vi "UMLEditor Main.vi"(1 "StartProject":string, 3 "StartTarget":string) -> ()   [LabVIEW 2012] (continued)
                        n1583 = call-dynamic "getBounds.vi"("reference"=w4053, "error in (no error)"=w4050) -> ("bounds"=w4048:T13, "error out"=w4051:errorcluster)  [unwired: 15 in, 1 out]
                        n1584 = Build Array(w4053) -> (w4047:refnum<class "AbstractNode.lvclass">[])
                        n1585 = Bundle By Name(cluster=w4055, "selcted"=UMLEditor_tooltype."Node", "SelectedNodes"=w4047, "dragStartBounds"=w4048, "dragStartPoint"=w4052, "lastMousePoint"=w4052, "newSelected"=TRUE, "toolType"=UMLEditor_tooltype."None", "tool"=UMLEditor_toolsType."CD_Select") -> (w4054:T7)
                        n1586 = call <resource>:"UMLEditor UpdatesToolbuttons.vi"() -> ()  [unwired: 6 in, 14 out]
                      }
                    }
                  }
                  frame True {
                    # "Added"
                    n1587 = case shown="\"AddNodeFromProjectTree+SyncAll\"" w4059 {
                      tunnel: [UMLEditor_statesType."Repaint" ("state") UMLEditor_statesType."SyncAll" ("state")] -> w4066
                      frame "AddNodeFromProjectTree", Default {
                      }
                      frame "AddNodeFromProjectTree+SyncAll" {
                      }
                    }
                    n1588 = To More Specific Class(target class=refnum<class "ClassNode.lvclass"> refnum ("reference"), reference=w4057) -> (specific class reference=w4056:refnum<class "ClassNode.lvclass">)  [unwired: 1 in, 1 out]
                    n1589 = call-dynamic "ExternalSetParam.vi"("reference"=w4056, "setParameter"=ExternalSetTypes."Name", "string"=w4067, "error in (no error)"=w4069) -> ("reference out"=w4063:refnum<class "ClassNode.lvclass">, "error out"=w4065:errorcluster)  [unwired: 14 in]
                    n1590 = call-dynamic "ExternalSetParam.vi"("reference"=w4063, "setParameter"=ExternalSetTypes."ClassPath", "error in (no error)"=w4065, "ClassPath"=w4060) -> ("reference out"=w4062:refnum<class "ClassNode.lvclass">, "error out"=w4064:errorcluster)  [unwired: 14 in]
                    n1591 = call-dynamic "getBounds.vi"("reference"=w4062, "error in (no error)"=w4064) -> ("reference out"=w4079:refnum<class "ClassNode.lvclass">, "bounds"=w4080:T13, "error out"=w4076:errorcluster)  [unwired: 15 in]
                    n1592 = Build Array(w4079) -> (w4071:refnum<class "ClassNode.lvclass">[])
                    n1593 = Bundle By Name(cluster=w4074, "selcted"=UMLEditor_tooltype."Node", "SelectedNodes"=w4071, "dragStartBounds"=w4080, "dragStartPoint"=w4070, "lastMousePoint"=w4070) -> (w4073:T7)
                    n1594 = call <resource>:"UMLEditor setDiagramInfo.vi"("error in (no error)"=w4076, "localVariablesIn"=w4073, "action"=enum16{"Name/Dir", "Unsaved", "Saved"}."Unsaved") -> ("localVariablesOut"=w4072:T7, "error out"=w4075:errorcluster)  [unwired: 2 in, 13 out]
                  }
                }
              }
            }
            n1595 = for {
              tunnel: w3971 -> [_]
              tunnel: w3946 -> [w4095] mode=indexing
              tunnel: [w4094] -> _
              n1596 = Close Reference(reference=w4095) -> (error out=w4094:errorcluster)  [unwired: 1 in]
            }
          }
          frame True {
            n1597 = call <resource>:"GDSError_ClearError.vi"("code"=1055, "error in (no error)"=w4098) -> ("error out"=w4097:errorcluster)  [unwired: 3 in, 14 out]
          }
        }
      }
      frame "AnalyseViInStateDiagram" {
        n1598 = Unbundle By Name(w4105) -> ("diagrams"=w4127:T39)
        n1599 = Unbundle By Name(w4105) -> ("menu"=w4120:refnum<k9>, "Action"=w4104:string)
        n1600 = property on="toolTab" class="TabCtl (strict)"("Disabled"=u8 0) -> ()  [unwired: 2 in, 2 out]
        n1601 = local write "Diagram"(0) -> ()
        n1602 = call <resource>:"UMLEditor UpdatesToolbuttons.vi"() -> ()  [unwired: 6 in, 14 out]
        n1603 = for {
          tunnel: w4127 -> [w4190] mode=indexing
          tunnel: "Untitled %d" -> [w4188]
          tunnel: [w4187] -> w4125 mode=indexing
          n1604 = Unbundle By Name(w4190) -> ("name"=w4189:string)
          n1605 = Scan From String(format string=w4188, input string=w4189) -> (output 1=w4187:i32)  [unwired: 2 in, 4 out]
        }
        n1606 = String To Path(string=w4104) -> (path=w4103:path)
        n1607 = Bundle By Name(cluster=T32 {"VI-Path"=path "", "ShowOption"=enum."Show Relative Path"} ("StateDiagramData"), "VI-Path"=w4103) -> (w4110:T32)
        n1608 = Unbundle By Name(w4105) -> ("grid"=w4112:refnum<class "Grid.lvclass">, "graphics"=w4111:refnum<class "Graphics.lvclass">)
        n1609 = Array Max & Min(array=w4125) -> (max value=w4124:i32)  [unwired: 3 out]
        n1610 = call <resource>:"StateDiagramGraph_Create.vi"("StateDiagramData"=w4110, "error in (no error)"=w4109) -> ("reference out"=w4115:refnum<class "StateDiagramGraph.lvclass">, "error out"=w4114:errorcluster)  [unwired: 2 in, 14 out]
        n1611 = property on="Picture" class="Pict"() -> (error out=w4102:errorcluster, "Visible"=w4101:bool)  [unwired: 2 in, 1 out]
        n1612 = call-dynamic "HandleRightClickMenuOption.vi"("reference"=w4115, "MenuOption"="Create New Diagram", "graphics"=w4111, "grid"=w4112, "error in (no error)"=w4114) -> ("reference out"=w4108:refnum<class "StateDiagramGraph.lvclass">, "Cancel"=w4107:bool, "error out"=w4106:errorcluster)  [unwired: 12 in]
        n1613 = property on="Picture" class="Pict"(error in=w4102, "Visible"=TRUE) -> ()  [unwired: 1 in, 2 out]
        n1614 = case shown="False" w4107 {
          tunnel: w4124 -> [w4153 _]
          tunnel: w4120 -> [w4135 _]
          tunnel: [w4134 w4184] -> w4119
          tunnel: [w4133 w4183] -> w4118
          tunnel: w4105 -> [w4132 w4183]
          tunnel: [UMLEditor_statesType."Repaint" ("state") UMLEditor_statesType."Idle" ("state")] -> w4117
          tunnel: w4108 -> [w4129 w4185]
          tunnel: w4106 -> [w4128 w4186]
          tunnel: w4101 -> [_ w4181]
          frame False {
            w4144 = diagramType."State" ("diagramType")
            n1615 = Increment(x=w4153) -> (x+1=w4151:i32)
            n1616 = local read "Help"() -> (w4145:bool)
            n1617 = Format Into String(format string="Untitled %d", w4151) -> (resulting string=w4147:string)  [unwired: 2 in, 1 out]
            n1618 = property on="Diagram" class="Ring (strict)"("Tip Strip"=w4147) -> ()  [unwired: 2 in, 2 out]
            n1619 = case shown="True" w4145 {
              tunnel: w4144 -> [_ w4157]
              frame False {
              }
              frame True {
                n1620 = case shown="\"State\"" w4157 {
                  tunnel: [ContextHelp_HelpTexts."ClassDiagram_Help" ("HelpText") ContextHelp_HelpTexts."UseCaseDiagram_Help" ("HelpText") ContextHelp_HelpTexts."SequenceDiagram_Help" ("HelpText") ContextHelp_HelpTexts."StateDiagram_Help" ("HelpText")] -> w4155
                  frame "Class", Default {
                  }
                  frame "UseCase" {
                  }
                  frame "Sequency" {
                  }
                  frame "State" {
                  }
                }
                n1621 = call <resource>:"ContextHelp_HelpTexts.vi"("HelpText (enum or string)"=w4155) -> ("HelpOut"=w4156:T57)  [unwired: 18 out]
                n1622 = call <resource>:"ContextHelp_SendMessageToPopUp.vi"("PopUpMessage"=w4156) -> ()  [unwired: 2 in, 17 out]
              }
            }
            n1623 = call <resource>:"UndoEngine.vi"("reference"=w4129, "Action"=enum16{"TakeSnapshot", "Undo", "Redo"}."TakeSnapshot", "Reset"=TRUE, "error in (no error)"=w4128, "menu"=w4135) -> ("error out"=w4130:errorcluster)  [unwired: 3 in, 11 out]
            n1624 = call <resource>:"UMLEditor addDiagram.vi"("graph"=w4129, "diagramType"=w4144, "name"=w4147, "saveDir"=path "", "unsaved(False)"=FALSE, "error in (no error)"=w4130, "localVariablesIn"=w4132) -> ("localVariablesOut"=w4148:T7, "error out"=w4149:errorcluster)  [unwired: 11 out]
            n1625 = case shown="\"Class\", Default" w4144 {
              tunnel: w4148 -> [w4163 w4167 w4171 w4176 w4180]
              tunnel: [w4162 w4166 w4170 w4175 w4179] -> w4142
              frame "None" {
                n1626 = Bundle By Name(cluster=w4163, "tool"=UMLEditor_toolsType."CD_Select") -> (w4162:T7)
              }
              frame "Sequency" {
                n1627 = property on="toolTab" class="TabCtl (strict)"("Value"=enum32{"Class", "Sequence", "UseCase"}."Sequence" ("toolTab")) -> ()  [unwired: 2 in, 2 out]
                n1628 = Bundle By Name(cluster=w4167, "tool"=UMLEditor_toolsType."SQD_Select") -> (w4166:T7)
              }
              frame "UseCase" {
                n1629 = property on="toolTab" class="TabCtl (strict)"("Value"=enum32{"Class", "Sequence", "UseCase"}."UseCase" ("toolTab")) -> ()  [unwired: 2 in, 2 out]
                n1630 = Bundle By Name(cluster=w4171, "tool"=UMLEditor_toolsType."UD_Select") -> (w4170:T7)
              }
              frame "State" {
                n1631 = property on="toolTab" class="TabCtl (strict)"("Value"=enum32{"Class", "Sequence", "UseCase", "State"}."State" ("toolTab")) -> ()  [unwired: 2 in, 2 out]
                n1632 = Bundle By Name(cluster=w4176, "tool"=UMLEditor_toolsType."STD_Select") -> (w4175:T7)
              }
              frame "Class", Default {
                n1633 = Bundle By Name(cluster=w4180, "tool"=UMLEditor_toolsType."CD_Select") -> (w4179:T7)
                n1634 = property on="toolTab" class="TabCtl (strict)"("Value"=enum32{"Class", "Sequence", "UseCase"}."Class" ("toolTab")) -> ()  [unwired: 2 in, 2 out]
              }
            }
            n1635 = Unbundle By Name(w4132) -> ("menu"=w4143:refnum<k9>)
            n1636 = Bundle By Name(cluster=w4142, "selectedEdge"=refnum<class "AbstractEdge.lvclass"> refnum, "SelectedNodes"=refnum<class "AbstractNode.lvclass">[] [], "selcted"=UMLEditor_tooltype."None", "toolType"=UMLEditor_tooltype."None") -> (w4133:T7)
            n1637 = call <resource>:"UMLEditor menuUpdates.vi"("menu"=w4143, "menuAction"=UMLEditor_MenuActionType."EnableSave", "error in (no error)"=w4149) -> ("error out"=w4134:errorcluster)  [unwired: 3 in, 13 out]
          }
          frame True {
            n1638 = property on="Picture" class="Pict"("Visible"=w4181) -> ()  [unwired: 2 in, 2 out]
            n1639 = call-dynamic "Destroy.vi"("reference"=w4185, "error in (no error)"=w4186) -> ("error out"=w4184:errorcluster)  [unwired: 16 in, 1 out]
          }
        }
      }
      frame "Copy", "CopyPaste" {
        n1640 = Unbundle By Name(w4192) -> ("SelectedNodes"=w4193:refnum<class "AbstractNode.lvclass">[], "menu"=w4196:refnum<k9>)
        n1641 = Array Size(array=w4193) -> (size(s)=w4197:i32)
        n1642 = case shown="1.." w4197 {
          tunnel: w4196 -> [_ w4213]
          tunnel: w4195 -> [w4201 w4205]
          tunnel: [w4201 w4206] -> w4194
          tunnel: w4193 -> [_ w4207]
          tunnel: w4192 -> [_ w4202]
          frame 0, Default {
          }
          frame 1.. {
            n1643 = call <resource>:"UMLEditor getDiagramInfo.vi"("localVariables"=w4202, "error in (no error)"=w4205) -> ("graph"=w4203:refnum<class "Graph.lvclass">, "error out"=w4204:errorcluster)  [unwired: 16 out]
            n1644 = call <resource>:"UMLEditor menuUpdates.vi"("menu"=w4213, "menuAction"=UMLEditor_MenuActionType."EnablePaste", "error in (no error)"=w4204) -> ("error out"=w4211:errorcluster)  [unwired: 3 in, 13 out]
            n1645 = call <resource>:"UMLEditor ClipBoard.vi"("menuAction"=UMLEditor_ClipBoardActionType."EmptyClipBoard", "error in (no error)"=w4211) -> ("error out"=w4209:errorcluster)  [unwired: 4 in, 13 out]
            n1646 = call <resource>:"UMLEditor ClipBoard.vi"("menuAction"=UMLEditor_ClipBoardActionType."InsertToClipBoard", "SelectedNodes"=w4207, "Graph"=w4203, "error in (no error)"=w4209) -> ("error out"=w4206:errorcluster)  [unwired: 2 in, 13 out]
          }
        }
        n1647 = case shown="\"CopyPaste\"" w4191 {
          tunnel: [UMLEditor_statesType."Paste" ("state") UMLEditor_statesType."Idle" ("state")] -> w4198
          frame "CopyPaste" {
          }
          frame Default {
          }
        }
      }
      frame "Paste" {
        n1648 = Unbundle By Name(w4215) -> ("graphics"=w4220:refnum<class "Graphics.lvclass">, "offset"=w4222:T12, "zoom"=w4221:dbl)
        n1649 = call <resource>:"UMLEditor getDiagramInfo.vi"("localVariables"=w4215, "error in (no error)"=w4219) -> ("graph"=w4216:refnum<class "Graph.lvclass">, "diagramType"=w4217:T11, "error out"=w4218:errorcluster)  [unwired: 15 out]
        n1650 = case shown="Default" w4217 {
          tunnel: [w4226 w4248] -> w4223
          tunnel: w4222 -> [_ w4245]
          tunnel: w4221 -> [_ w4244]
          tunnel: w4220 -> [_ w4243]
          tunnel: w4218 -> [w4226 w4235]
          tunnel: w4216 -> [_ w4234]
          tunnel: w4215 -> [w4225 w4233]
          tunnel: [w4225 w4232] -> w4214
          frame "None" {
          }
          frame Default {
            w4242 = cluster{dbl, dbl} {0.0, 0.0} ("lower limit")
            n1651 = property on="Picture" class="Pict"() -> ("Mouse"=w4237:T42)  [unwired: 2 in, 2 out]
            n1652 = Unbundle By Name(w4237) -> ("Mouse Position"=w4247:cluster{"X":i32, "Y":i32})
            n1653 = Add(x=w4247, y=w4245) -> (x+y=w4246:T12)
            n1654 = Divide(x=w4246, y=w4244) -> (x/y=w4228:T12)
            n1655 = call <resource>:"getScreenBounds.vi"("reference"=w4243, "error in (no error)"=w4235) -> ("bounds"=w4241:T13, "error out"=w4236:errorcluster)  [unwired: 16 out]
            n1656 = Unbundle By Name(w4241) -> ("width"=w4240:dbl, "height"=w4239:dbl)
            n1657 = Bundle(cluster=w4242, w4240, w4239) -> ()  [unwired: 1 out]
            n1658 = In Range and Coerce(upper limit=w4228, x=w4228, lower limit=w4242) -> (coerced(x)=w4238:T12)  [unwired: 1 out]
            n1659 = call <resource>:"UMLEditor ClipBoard.vi"("menuAction"=UMLEditor_ClipBoardActionType."PasteContentAtPos", "Pos"=w4238, "Graph"=w4234, "error in (no error)"=w4236, "LimitPasteToAllowedLocations(True)"=FALSE) -> ("PastedNodes"=w4231:refnum<class "AbstractNode.lvclass">[], "error out"=w4248:errorcluster)  [unwired: 2 in, 11 out]
            n1660 = Array Size(array=w4231) -> (size(s)=w4229:i32)
            n1661 = case shown="0" w4229 {
              tunnel: [UMLEditor_tooltype."Node" ("selcted") UMLEditor_tooltype."None" ("selcted")] -> w4230
              frame Default {
              }
              frame 0 {
              }
            }
            n1662 = Bundle By Name(cluster=w4233, "selcted"=w4230, "SelectedNodes"=w4231) -> (w4232:T7)
          }
        }
      }
      frame "Export" {
        w4253 = 0.0 ("y")
        w4252 = 5.0  # borderRoundPicture
        w4287 = 1.0 ("scaleX")
        n1663 = Unbundle By Name(w4260) -> ("graphics"=w4290:refnum<class "Graphics.lvclass">)
        n1664 = Unbundle By Name(w4260) -> ("exportype"=w4259:T14)
        n1665 = Unbundle By Name(w4260) -> ("grid"=w4282:refnum<class "Grid.lvclass">)
        n1666 = call-dynamic "clone.vi"("reference"=w4290, "error in (no error)"=w4289) -> ("clonedObjectRef"=w4288:refnum<class "Graphics.lvclass">, "error out"=w4286:errorcluster)  [unwired: 15 in, 1 out]
        n1667 = call <resource>:"scale.vi"("reference"=w4288, "scaleX"=w4287, "scaleY"=w4287, "error in (no error)"=w4286) -> ("reference out"=w4278:refnum<class "Graphics.lvclass">, "error out"=w4279:errorcluster)  [unwired: 14 out]
        n1668 = call <resource>:"resetPicture.vi"("reference"=w4278, "error in (no error)"=w4279) -> ("reference out"=w4277:refnum<class "Graphics.lvclass">, "error out"=w4276:errorcluster)  [unwired: 16 out]
        n1669 = call <resource>:"UMLEditor getDiagramInfo.vi"("localVariables"=w4260, "error in (no error)"=w4276) -> ("graph"=w4284:refnum<class "Graph.lvclass">, "name"=w4257:string, "saveDir"=w4258:path, "error out"=w4285:errorcluster)  [unwired: 14 out]
        n1670 = call-dynamic "getBounds.vi"("reference"=w4284, "graphics"=w4277, "error in (no error)"=w4285) -> ("reference out"=w4283:refnum<class "Graph.lvclass">, "bounds"=w4270:T13, "error out"=w4275:errorcluster)  [unwired: 14 in]
        n1671 = Unbundle By Name(w4270) -> ("width"=w4268:dbl, "height"=w4269:dbl)
        n1672 = Unbundle By Name(w4270) -> ("x"=w4274:dbl, "y"=w4271:dbl)
        n1673 = Subtract(x=w4274, y=w4253) -> (x-y=w4273:dbl)
        n1674 = Subtract(x=w4271, y=w4253) -> (x-y=w4272:dbl)
        n1675 = Add(x=w4268, y=w4269) -> (x+y=w4267:dbl)
        n1676 = Greater Than 0?(x=w4267) -> (x > 0?=w4266:bool)
        n1677 = call <resource>:"setOffset.vi"("reference"=w4277, "offsetX"=w4273, "offsetY"=w4272, "error in (no error)"=w4275) -> ("reference out"=w4265:refnum<class "Graphics.lvclass">, "error out"=w4254:errorcluster)  [unwired: 14 out]
        n1678 = Multiply(x=w4252, y=2.0) -> (x*y=w4261:dbl)
        n1679 = call-dynamic "draw.vi"("reference"=w4283, "graphics"=w4265, "grid"=w4282, "error in (no error)"=w4254, "SelectedNodes"=refnum<class "AbstractNode.lvclass">[] [], "HideOverLays(False)"=TRUE) -> ("NodesBounds"=w4281:T13, "error out"=w4263:errorcluster)  [unwired: 10 in, 2 out]
        n1680 = case shown="True" w4266 {
          tunnel: w4281 -> [_ _]
          tunnel: w4270 -> [_ w4314]
          tunnel: w4265 -> [_ w4315]
          tunnel: w4263 -> [w4292 w4300]
          tunnel: [w4292 w4300] -> w4264
          tunnel: w4261 -> [_ w4304]
          tunnel: w4259 -> [_ w4299]
          tunnel: w4259 -> [_ w4307]
          tunnel: w4258 -> [_ w4306]
          tunnel: w4257 -> [_ w4301]
          tunnel: w4252 -> [_ w4294]
          frame False {
          }
          frame True {
            n1681 = Match Pattern(string=w4301, regular expression="[.][~.]+$") -> (before substring=w4302:string)  [unwired: 4 out]
            n1682 = Unbundle By Name(w4314) -> ("x"=w4297:dbl, "y"=w4295:dbl, "width"=w4312:dbl, "height"=w4310:dbl)
            n1683 = case shown="\"None\", Default" w4307 {
              tunnel: w4306 -> [_ w4323 w4328 _]
              tunnel: w4302 -> [_ w4321 w4326 _]
              tunnel: [path "" ("Not A Path Constant") w4319 w4324 path "" ("Not A Path Constant")] -> w4305
              frame "None", Default {
              }
              frame "png" {
                n1684 = Concatenate Strings(w4321, ".png" ("string")) -> (w4322:string)
                n1685 = Build Path(base path=w4323, name or relative path=w4322) -> (appended path=w4319:path)
              }
              frame "jpg" {
                n1686 = Concatenate Strings(w4326, ".jpg" ("string")) -> (w4327:string)
                n1687 = Build Path(base path=w4328, name or relative path=w4327) -> (appended path=w4324:path)
              }
              frame "Printer" {
              }
            }
            n1688 = Subtract(x=w4297, y=w4294) -> (x-y=w4296:dbl)
            n1689 = Subtract(x=w4295, y=w4294) -> (x-y=w4293:dbl)
            n1690 = Add(x=w4312, y=w4304) -> (x+y=w4311:dbl)
            n1691 = Add(x=w4310, y=w4304) -> (x+y=w4309:dbl)
            n1692 = Bundle By Name(cluster=T13 {"x"=0.0, "y"=0.0, "width"=0.0, "height"=0.0} ("bounds"), "x"=w4296, "y"=w4293, "width"=w4311, "height"=w4309) -> (w4308:T13)
            n1693 = call <resource>:"UMLEditor export.vi"("graphics"=w4315, "bounds"=w4308, "exportype"=w4299, "fileName"=w4305, "error in (no error)"=w4300) -> ("error out"=w4298:errorcluster)  [unwired: 14 out]
            n1694 = case shown="\"Printer\"" w4299 {
              tunnel: w4298 -> [_ w4316]
              frame "None", Default {
              }
              frame "Printer" {
                n1695 = case shown="Error" w4316 {
                  frame No Error {
                  }
                  frame Error {
                    n1696 = One Button Dialog(message="Error while printing\nCheck the default printer settings.") -> ()  [unwired: 2 out]
                  }
                }
              }
            }
          }
        }
        n1697 = call-dynamic "Destroy.vi"("reference"=w4265, "error in (no error)"=w4264) -> ("error out"=w4280:errorcluster)  [unwired: 16 in, 1 out]
      }
      frame "EditSelected" {
        n1698 = Unbundle By Name(w4332) -> ("selcted"=w4343:T9, "selectedEdge"=w4337:refnum<class "AbstractEdge.lvclass">, "SelectedNodes"=w4341:refnum<class "AbstractNode.lvclass">[])
        n1699 = Unbundle By Name(w4332) -> ("graphics"=w4331:refnum<class "Graphics.lvclass">, "grid"=w4330:refnum<class "Grid.lvclass">)
        n1700 = call <resource>:"UMLEditor getDiagramInfo.vi"("localVariables"=w4332, "error in (no error)"=w4340) -> ("graph"=w4338:refnum<class "Graph.lvclass">, "diagramType"=w4335:T11, "error out"=w4339:errorcluster)  [unwired: 15 out]
        n1701 = Bundle By Name(cluster=w4332, "newSelected"=FALSE) -> (w4334:T7)
        n1702 = case shown="\"Node\"" w4343 {
          tunnel: w4339 -> [w4349 w4379 w4447]
          tunnel: [w4347 w4380 w4441] -> w4342
          tunnel: w4341 -> [_ w4368 _]
          tunnel: w4338 -> [w4348 w4375 w4445]
          tunnel: w4337 -> [_ _ w4444]
          tunnel: w4334 -> [w4346 w4366 w4443]
          tunnel: [w4345 w4370 w4442] -> w4336
          tunnel: w4335 -> [w4350 _ _]
          tunnel: w4331 -> [_ w4363 _]
          tunnel: w4330 -> [_ w4362 _]
          frame "None", Default {
            n1703 = case shown="Default" w4350 {
              tunnel: w4349 -> [w4352 w4361]
              tunnel: w4348 -> [_ w4355]
              tunnel: [w4352 w4358] -> w4347
              tunnel: w4346 -> [w4351 w4357]
              tunnel: [w4351 w4356] -> w4345
              frame Default {
              }
              frame "State" {
                n1704 = To More Specific Class(target class=refnum<class "StateDiagramGraph.lvclass"> refnum ("reference out"), reference=w4355) -> (specific class reference=w4353:refnum<class "StateDiagramGraph.lvclass">)  [unwired: 1 in, 1 out]
                n1705 = call-dynamic "editDialog.vi"("reference"=w4353, "error in (no error)"=w4361) -> ("error out"=w4359:errorcluster)  [unwired: 15 in, 2 out]
                n1706 = call <resource>:"UMLEditor setDiagramInfo.vi"("error in (no error)"=w4359, "localVariablesIn"=w4357, "action"=enum16{"Name/Dir", "Unsaved", "Saved"}."Unsaved") -> ("localVariablesOut"=w4356:T7, "error out"=w4358:errorcluster)  [unwired: 2 in, 13 out]
              }
            }
          }
          frame "Node" {
            n1707 = Index Array(array=w4368) -> (element=w4365:refnum<class "AbstractNode.lvclass">)  [unwired: 1 in]
            n1708 = call-dynamic "contains.vi"("reference"=w4375, "node"=w4365, "nodeType(Empty=AllNodeTypesAllaowed)"=string[] ["PackageNode$", "SystemNode$"], "error in (no error)"=w4379) -> ("contains"=w4374:bool, "container"=w4373:refnum<class "AbstractNode.lvclass">, "error out"=w4378:errorcluster)  [unwired: 12 in, 1 out]
            n1709 = call-dynamic "editDialog.vi"("reference"=w4365, "insidePackageNode"=w4374, "error in (no error)"=w4378) -> ("reference out"=w4372:refnum<class "AbstractNode.lvclass">, "changeConnection"=w4377:T61, "cancel"=w4371:bool, "error out"=w4376:errorcluster)  [unwired: 13 in]
            n1710 = Build Array(w4365) -> (w4364:refnum<class "AbstractNode.lvclass">[])
            n1711 = Bundle By Name(cluster=w4366, "SelectedNodes"=w4364) -> (w4367:T7)
            n1712 = case shown="False" w4371 {
              tunnel: [w4387 w4439] -> w4380
              tunnel: w4377 -> [w4394 _]
              tunnel: w4376 -> [w4393 w4439]
              tunnel: w4375 -> [w4383 _]
              tunnel: w4373 -> [w4392 _]
              tunnel: w4372 -> [w4391 _]
              tunnel: w4367 -> [w4386 w4438]
              tunnel: [w4385 w4438] -> w4370
              tunnel: w4363 -> [w4382 _]
              tunnel: w4362 -> [w4381 _]
              frame False {
                n1713 = case shown="\"Connect\"" w4394 {
                  tunnel: w4393 -> [w4397 w4405 w4410]
                  tunnel: w4392 -> [_ w4404 w4431]
                  tunnel: w4391 -> [w4396 w4402 w4408]
                  tunnel: [w4397 w4399 w4422] -> w4390
                  tunnel: [w4395 _ _] -> w4384
                  tunnel: w4383 -> [_ w4398 w4426]
                  tunnel: w4382 -> [_ _ w4425]
                  tunnel: w4381 -> [_ _ w4424]
                  frame "NA", Default {
                    n1714 = Build Array(w4396) -> (w4395:refnum<class "AbstractNode.lvclass">[])
                  }
                  frame "Connect" {
                    n1715 = call-dynamic "addChild.vi"("reference"=w4404, "node"=w4402, "error in (no error)"=w4405) -> ("reference out"=w4401:refnum<class "AbstractNode.lvclass">, "error out"=w4403:errorcluster)  [unwired: 15 in]
                    n1716 = call-dynamic "setParent.vi"("reference"=w4402, "node"=w4401, "error in (no error)"=w4403) -> ("error out"=w4400:errorcluster)  [unwired: 15 in, 1 out]
                    n1717 = call-dynamic "RearrangeNodes.vi"("reference in"=w4398, "error in (no error)"=w4400) -> ("error out"=w4399:errorcluster)  [unwired: 16 in, 1 out]
                  }
                  frame "DisConnect" {
                    n1718 = call-dynamic "GetParentsRecurivly.vi"("reference"=w4408, "error in (no error)"=w4410) -> ("Parents"=w4407:refnum<class "AbstractNode.lvclass">[], "error out"=w4409:errorcluster)  [unwired: 15 in, 1 out]
                    n1719 = call-dynamic "removeChild.vi"("reference"=w4431, "node"=w4408, "error in (no error)"=w4409) -> ("reference out"=w4427:refnum<class "AbstractNode.lvclass">, "error out"=w4430:errorcluster)  [unwired: 15 in]
                    n1720 = call-dynamic "setParent.vi"("reference"=w4408, "node"=refnum<class "AbstractNode.lvclass"> refnum, "error in (no error)"=w4430) -> ("error out"=w4428:errorcluster)  [unwired: 15 in, 1 out]
                    n1721 = call-dynamic "layout.vi"("reference"=w4427, "graph"=w4426, "graphics"=w4425, "grid"=w4424, "error in (no error)"=w4428) -> ("error out"=w4423:errorcluster)  [unwired: 13 in, 1 out]
                    n1722 = Delete From Array(array=w4407) -> (deleted portion=w4406:refnum<class "AbstractNode.lvclass">)  [unwired: 2 in, 1 out]
                    n1723 = call-dynamic "getBounds.vi"("reference"=w4406, "error in (no error)"=w4423) -> ("bounds"=w4420:T13, "error out"=w4421:errorcluster)  [unwired: 15 in, 1 out]
                    n1724 = call <resource>:"Rectangel GetRectInfo.vi"("bounds"=w4420) -> ("maxX"=w4418:dbl)  [unwired: 1 in, 17 out]
                    n1725 = call-dynamic "getBounds.vi"("reference"=w4408, "error in (no error)"=w4421) -> ("reference out"=w4413:refnum<class "AbstractNode.lvclass">, "bounds"=w4419:T13, "error out"=w4412:errorcluster)  [unwired: 15 in]
                    n1726 = Unbundle By Name(w4419) -> ("x"=w4417:dbl)
                    n1727 = Subtract(x=w4418, y=w4417) -> (x-y=w4416:dbl)
                    n1728 = Add(x=10.0, y=w4416) -> (x+y=w4414:dbl)
                    n1729 = Greater Or Equal To 0?(x=w4414) -> (x >= 0?=w4411:bool)
                    n1730 = case shown="True" w4411 {
                      tunnel: [w4432 w4437] -> w4422
                      tunnel: w4414 -> [_ w4436]
                      tunnel: w4413 -> [_ w4435]
                      tunnel: w4412 -> [w4432 w4434]
                      frame False {
                      }
                      frame True {
                        n1731 = call-dynamic "translate.vi"("reference"=w4435, "dx"=w4436, "dy"=0.0, "error in (no error)"=w4434) -> ("error out"=w4437:errorcluster)  [unwired: 14 in, 1 out]
                      }
                    }
                  }
                }
                n1732 = call-dynamic "layout.vi"("reference"=w4383, "LayoutNodes(Empty=All)"=w4384, "error in (no error)"=w4390) -> ("error out"=w4388:errorcluster)  [unwired: 15 in, 1 out]
                n1733 = call <resource>:"UMLEditor setDiagramInfo.vi"("error in (no error)"=w4388, "localVariablesIn"=w4386, "action"=enum16{"Name/Dir", "Unsaved", "Saved"}."Unsaved") -> ("localVariablesOut"=w4385:T7, "error out"=w4387:errorcluster)  [unwired: 2 in, 13 out]
              }
              frame True {
              }
            }
          }
          frame "Edge" {
            n1734 = call-dynamic "editDialog.vi"("reference"=w4444, "error in (no error)"=w4447) -> ("cancel"=w4440:bool, "error out"=w4446:errorcluster)  [unwired: 15 in, 1 out]
            n1735 = case shown="True" w4440 {
              tunnel: w4446 -> [w4455 w4461]
              tunnel: w4445 -> [w4454 _]
              tunnel: w4443 -> [w4452 w4460]
              tunnel: [w4451 w4460] -> w4442
              tunnel: [w4449 w4461] -> w4441
              frame False {
                n1736 = case shown="False" FALSE ("Case Constant\n(See Context Help) 4") {
                  tunnel: w4455 -> [w4456 w4459]
                  tunnel: w4454 -> [_ w4458]
                  tunnel: [w4456 w4457] -> w4450
                  frame False {
                  }
                  frame True {
                    n1737 = call-dynamic "layout.vi"("reference"=w4458, "error in (no error)"=w4459) -> ("error out"=w4457:errorcluster)  [unwired: 16 in, 1 out]
                  }
                }
                n1738 = call <resource>:"UMLEditor setDiagramInfo.vi"("error in (no error)"=w4450, "localVariablesIn"=w4452, "action"=enum16{"Name/Dir", "Unsaved", "Saved"}."Unsaved") -> ("localVariablesOut"=w4451:T7, "error out"=w4449:errorcluster)  [unwired: 2 in, 13 out]
              }
              frame True {
              }
            }
          }
        }
      }
      frame "RemoveSelected" {
        # "if aggregartion, check if we should remove ClassRef Attribute"
        n1739 = Unbundle By Name(w4470) -> ("selcted"=w4466:T9, "selectedEdge"=w4472:refnum<class "AbstractEdge.lvclass">, "SelectedNodes"=w4471:refnum<class "AbstractNode.lvclass">[], "Don'tDeleteChildren"=w4462:bool)
        n1740 = call <resource>:"UMLEditor getDiagramInfo.vi"("localVariables"=w4470, "error in (no error)"=w4474) -> ("graph"=w4473:refnum<class "Graph.lvclass">, "error out"=w4463:errorcluster)  [unwired: 16 out]
        n1741 = case shown="\"Node\"" w4466 {
          tunnel: [w4487 w4495 w4515] -> w4468
          tunnel: w4473 -> [_ w4494 w4517]
          tunnel: w4463 -> [w4487 w4492 w4514]
          tunnel: w4472 -> [_ w4493 _]
          tunnel: w4471 -> [_ _ w4516]
          tunnel: w4462 -> [_ _ w4513]
          frame "None", Default {
          }
          frame "Edge" {
            n1742 = call <resource>:"UMLEditor ShowAggregationDialog.vi"("graph"=w4494, "ClassAggregation"=w4493, "error in (no error)"=w4492) -> ("Base class.bounds"=w4489:T13, "Remove"=w4490:bool, "StartEndNodes"=w4488:T59, "error out"=w4491:errorcluster)  [unwired: 13 out]
            n1743 = stacked-sequence {
              tunnel: [w4502] -> w4495
              tunnel: w4494 -> [w4501]
              tunnel: w4493 -> [w4500]
              tunnel: w4492 -> [w4499]
              tunnel: w4491 -> [_]
              tunnel: w4490 -> [w4498]
              tunnel: w4489 -> [w4497]
              tunnel: w4488 -> [w4496]
              frame #0 {
                n1744 = case shown="True" w4498 {
                  tunnel: w4497 -> [_ w4509]
                  tunnel: w4496 -> [_ w4503]
                  frame False {
                  }
                  frame True {
                    n1745 = Unbundle(w4509) -> ("x"=w4508:dbl, "y"=w4504:dbl, "width"=w4507:dbl)  [unwired: 1 out]
                    n1746 = Add(x=w4508, y=w4507) -> (x+y=w4506:dbl)
                    n1747 = Bundle(cluster=cluster{"X":i32, "Y":i32} {"X"=100, "Y"=100} ("Mouse Position"), "X"=w4506, "Y"=w4504) -> (w4505:cluster{"X":i32, "Y":i32})
                    n1748 = call <resource>:"UMLEditor_AggregationClusterDialogControl.vi"("Position"=w4505, "Action(SelectSelect)"=T22."DeleteAggregation", "StartEndNodesIn"=w4503) -> ()  [unwired: 6 in, 11 out]
                  }
                }
                n1749 = call-dynamic "removeEdge.vi"("reference"=w4501, "edge"=w4500, "error in (no error)"=w4499) -> ("error out"=w4502:errorcluster)  [unwired: 15 in, 1 out]
              }
            }
          }
          frame "Node" {
            n1750 = Not(x=w4513) -> (.not. x?=w4512:bool)
            n1751 = for {
              tunnel: w4517 -> [w4522]
              tunnel: w4516 -> [w4521] mode=indexing
              shift-right: [w4520] -> w4515
              shift-left: w4514 -> [w4519]
              tunnel: w4512 -> [w4518]
              n1752 = call-dynamic "removeNode.vi"("reference"=w4522, "node"=w4521, "RemoveChildrenIfAny(False)"=w4518, "error in (no error)"=w4519) -> ("error out"=w4520:errorcluster)  [unwired: 14 in, 1 out]
            }
          }
        }
        n1753 = Bundle By Name(cluster=w4470, "selcted"=UMLEditor_tooltype."None") -> (w4465:T7)
        n1754 = case shown="\"Node\", \"Edge\"" w4466 {
          tunnel: w4468 -> [w4477 w4485]
          tunnel: [w4477 w4484] -> w4467
          tunnel: [w4476 w4481] -> w4464
          tunnel: w4465 -> [w4476 w4483]
          frame "None", Default {
          }
          frame "Node", "Edge" {
            n1755 = call <resource>:"UMLEditor setDiagramInfo.vi"("error in (no error)"=w4485, "localVariablesIn"=w4483, "action"=enum16{"Name/Dir", "Unsaved", "Saved"}."Unsaved") -> ("localVariablesOut"=w4482:T7, "error out"=w4484:errorcluster)  [unwired: 2 in, 13 out]
            n1756 = Bundle By Name(cluster=w4482, "SelectedNodes"=refnum<class "AbstractNode.lvclass">[] [], "selectedEdge"=refnum<class "AbstractEdge.lvclass"> refnum, "modified"=TRUE) -> (w4481:T7)
          }
        }
      }
      frame "Save" {
        w4526 = UMLEditor_statesType."Close" ("x")
        n1757 = Unbundle By Name(w4528) -> ("saveAs"=w4530:bool)
        n1758 = call <resource>:"UMLEditor getDiagramInfo.vi"("localVariables"=w4528, "error in (no error)"=w4550) -> ("graph"=w4548:refnum<class "Graph.lvclass">, "name"=w4540:string, "diagramType"=w4547:T11, "saveDir"=w4537:path, "error out"=w4546:errorcluster)  [unwired: 13 out]
        n1759 = Empty String/Path?(string/path=w4537) -> (empty?=w4525:bool)
        n1760 = File/Directory Info(path=w4537, error in=w4546) -> (directory=w4535:bool, error out=w4544:errorcluster)  [unwired: 5 out]
        n1761 = call <resource>:"File_ApplicationPaths.vi"("PathName"=UMLEditor_StoredPathes."LastSearchPath" ("UMLPathes")) -> ("Path Out"=w4523:path)  [unwired: 3 in, 15 out]
        n1762 = Bundle By Name(cluster=w4528, "saveAs"=FALSE) -> (w4529:T7)
        n1763 = Compound Arithmetic op=AND(invert w4530, invert w4525, w4535) -> (w4536:bool)
        n1764 = case shown="False" w4536 {
          tunnel: w4544 -> [w4568 w4591]
          tunnel: [w4567 w4591] -> w4543
          tunnel: [w4562 w4593] -> w4542
          tunnel: w4537 -> [w4553 w4593]
          tunnel: [w4561 w4592] -> w4541
          tunnel: w4540 -> [w4560 w4592]
          tunnel: w4529 -> [w4566 w4594]
          tunnel: [w4565 w4594] -> w4539
          tunnel: [w4556 FALSE ("cancelled")] -> w4538
          tunnel: w4525 -> [w4554 _]
          tunnel: w4523 -> [w4551 _]
          frame False {
            (unwired) T58."new or existing file" ("select mode (2)")
            n1765 = Select(t=w4551, s=w4554, f=w4553) -> (s? t:f=w4552:path)
            n1766 = File Dialog(6:"*.uml" ("pattern"), 7:"Select file name" ("prompt"), 11:w4552) -> (1:w4557:bool, 2:w4559:bool, 3:w4558:path)  [unwired: 1 in, 4 out]
            n1767 = case shown="True" w4559 {
              tunnel: [w4569 w4572] -> w4556
              tunnel: w4557 -> [w4569 _]
              tunnel: w4558 -> [w4570 w4571]
              tunnel: [w4570 w4571] -> w4555
              frame False {
              }
              frame True {
                n1768 = Two Button Dialog(message="This file already exists.\nDo you want to overwrite it?", 1:"No" ("F button name (\"Cancel\")"), 2:"Yes" ("T button name (\"OK\")")) -> (T button?=w4573:bool)
                n1769 = case shown="True" w4573 {
                  tunnel: w4571 -> [_ w4577]
                  frame False {
                  }
                  frame True {
                    n1770 = Delete(path (use dialog)=w4577) -> ()  [unwired: 1 in, 6 out]
                  }
                }
                n1771 = Not(x=w4573) -> (.not. x?=w4572:bool)
              }
            }
            n1772 = case shown="True" w4556 {
              tunnel: w4568 -> [w4584 w4586]
              tunnel: [w4583 w4586] -> w4567
              tunnel: w4566 -> [w4582 w4589]
              tunnel: [w4581 w4589] -> w4565
              tunnel: w4555 -> [w4580 _]
              tunnel: [w4579 w4588] -> w4562
              tunnel: [w4578 w4587] -> w4561
              tunnel: w4552 -> [_ w4588]
              tunnel: w4560 -> [_ w4587]
              frame False {
                n1773 = Strip Path(path=w4580) -> (stripped path=w4579:path, name=w4578:string)
                n1774 = call <resource>:"UMLEditor setDiagramInfo.vi"("name"=w4578, "saveDir"=w4579, "error in (no error)"=w4584, "localVariablesIn"=w4582, "action"=enum16{"Name/Dir", "Unsaved", "Saved"}."Name/Dir") -> ("localVariablesOut"=w4581:T7, "error out"=w4583:errorcluster)  [unwired: 13 out]
              }
              frame True {
              }
            }
          }
          frame True {
          }
        }
        n1775 = Equal?(x=w4526, y=w4534) -> (x = y?=w4533:bool)
        n1776 = case shown="False" w4538 {
          tunnel: [w4598 w4627] -> w4549
          tunnel: w4548 -> [w4611 _]
          tunnel: w4547 -> [w4610 _]
          tunnel: w4543 -> [w4609 w4627]
          tunnel: w4539 -> [w4608 w4626]
          tunnel: [w4607 w4626] -> w4545
          tunnel: w4542 -> [w4603 _]
          tunnel: w4541 -> [w4606 _]
          frame False {
            n1777 = Build Path(base path=w4603, name or relative path=w4606) -> (appended path=w4602:path)
            n1778 = Path To String(path=w4602) -> (string=w4604:string)
            n1779 = call-dynamic "saveGraph.vi"("reference"=w4611, "filePath"=w4602, "diagramType"=w4610, "error in (no error)"=w4609) -> ("reference out"=w4596:refnum<class "Graph.lvclass">, "succeeded"=w4605:bool, "error out"=w4601:errorcluster)  [unwired: 13 in]
            n1780 = property on="Diagram" class="Ring (strict)"("Tip Strip"=w4604) -> ()  [unwired: 2 in, 2 out]
            n1781 = case shown="False" w4605 {
              tunnel: w4608 -> [w4613 w4616]
              tunnel: [w4613 w4617] -> w4607
              tunnel: w4601 -> [w4614 w4624]
              tunnel: [w4614 w4622] -> w4597
              tunnel: w4602 -> [_ w4619]
              tunnel: [w4612 w4615] -> w4595
              frame False {
                n1782 = Unbundle By Name(w4613) -> ("menu"=w4612:refnum<k9>)
              }
              frame True {
                n1783 = call <resource>:"UMLEditor setDiagramInfo.vi"("error in (no error)"=w4624, "localVariablesIn"=w4616, "action"=enum16{"Name/Dir", "Unsaved", "Saved"}."Saved") -> ("localVariablesOut"=w4617:T7, "error out"=w4623:errorcluster)  [unwired: 2 in, 13 out]
                n1784 = Unbundle By Name(w4616) -> ("menu"=w4615:refnum<k9>)
                n1785 = Path To String(path=w4619) -> (string=w4620:string)
                n1786 = call <resource>:"UMLEditor menuUpdates.vi"("menu"=w4615, "menuAction"=UMLEditor_MenuActionType."AddRecentFile", "item"=w4620, "addfirst(false)"=TRUE, "error in (no error)"=w4623) -> ("error out"=w4622:errorcluster)  [unwired: 1 in, 13 out]
              }
            }
            n1787 = call <resource>:"UndoEngine.vi"("reference"=w4596, "Action"=enum16{"TakeSnapshot", "Undo", "Redo"}."TakeSnapshot", "Reset"=TRUE, "error in (no error)"=w4597, "menu"=w4595) -> ("error out"=w4598:errorcluster)  [unwired: 3 in, 11 out]
          }
          frame True {
          }
        }
        n1788 = Select(t=w4526, s=w4533, f=UMLEditor_statesType."Repaint" ("state")) -> (s? t:f=w4531:T8)
      }
      frame "Open" {
        n1789 = Unbundle By Name(w4634) -> ("diagrams"=w4631:T39, "file"=w4637:path)
        n1790 = call <resource>:"UMLEditor getDiagramInfo.vi"("localVariables"=w4634, "error in (no error)"=w4651) -> ("graph"=w4650:refnum<class "Graph.lvclass">, "unsaved"=w4644:bool, "saveDir"=w4645:path, "error out"=w4648:errorcluster)  [unwired: 14 out]
        n1791 = Empty String/Path?(string/path=w4637) -> (empty?=w4638:bool)
        n1792 = Empty String/Path?(string/path=w4645) -> (empty?=w4643:bool)
        n1793 = call <resource>:"File_ApplicationPaths.vi"("PathName"=UMLEditor_StoredPathes."LastSearchPath" ("UMLPathes")) -> ("Path Out"=w4632:path)  [unwired: 3 in, 15 out]
        n1794 = case shown="False" w4638 {
          tunnel: [w4657 w4666] -> w4649
          tunnel: [w4659 w4665] -> w4647
          tunnel: w4645 -> [_ w4662]
          tunnel: w4637 -> [w4659 _]
          tunnel: "*.uml)\u0000*.uml;\u0000Backup files (*.bak)\u0000*.bak\u0000\u0000" ("pattern") -> [_ w4664]
          tunnel: w4632 -> [_ w4660]
          frame False {
            n1795 = File/Directory Info(path=w4659) -> (size=w4656:i64)  [unwired: 1 in, 6 out]
            n1796 = To Long Integer(number=w4656) -> (32bit integer=w4658:i32)
            n1797 = Greater Than 0?(x=w4658) -> (x > 0?=w4657:bool)
          }
          frame True {
            (unwired) T58."existing file" ("select mode (2)")
            n1798 = Empty String/Path?(string/path=w4662) -> (empty?=w4663:bool)
            n1799 = Select(t=w4660, s=w4663, f=w4662) -> (s? t:f=w4661:path)
            n1800 = File Dialog(6:w4664, 7:"Select file-name" ("prompt"), 11:w4661) -> (1:w4667:bool, 2:w4668:bool, 3:w4665:path)  [unwired: 1 in, 4 out]
            n1801 = Compound Arithmetic op=AND(w4668, invert w4667) -> (w4666:bool)
          }
        }
        n1802 = for {
          tunnel: w4631 -> [w4655] mode=indexing
          tunnel: [w4652] -> w4630 mode=indexing
          n1803 = Unbundle By Name(w4655) -> ("saveDir"=w4654:path, "name"=w4653:string)
          n1804 = Build Path(base path=w4654, name or relative path=w4653) -> (appended path=w4652:path)
        }
        n1805 = Compound Arithmetic op=AND(invert w4644, w4643) -> (w4642:bool)
        n1806 = Bundle By Name(cluster=w4634, "file"=path "", "Sync"=FALSE) -> (w4640:T7)
        n1807 = case shown="True" w4649 {
          tunnel: w4650 -> [_ _]
          tunnel: w4648 -> [w4672 w4684]
          tunnel: w4647 -> [_ w4675]
          tunnel: w4640 -> [w4671 w4683]
          tunnel: [w4672 w4681] -> w4646
          tunnel: w4642 -> [_ w4682]
          tunnel: [w4671 w4680] -> w4641
          tunnel: [UMLEditor_statesType."Idle" ("state") w4679] -> w4636
          tunnel: w4634 -> [_ w4678]
          tunnel: w4630 -> [_ w4674]
          frame False {
          }
          frame True {
            n1808 = Unbundle By Name(w4678) -> ("graphics"=w4676:refnum<class "Graphics.lvclass">, "grid"=w4677:refnum<class "Grid.lvclass">)
            n1809 = Search 1D Array(1D array=w4674, element=w4675) -> (index of element=w4673:i32)  [unwired: 1 in]
            n1810 = case shown="-1" w4673 {
              selector: w4673 -> [w4685 _]
              tunnel: w4684 -> [w4688 w4689]
              tunnel: w4683 -> [w4687 w4704]
              tunnel: w4682 -> [_ w4698]
              tunnel: [w4688 w4697] -> w4681
              tunnel: [w4687 w4696] -> w4680
              tunnel: [UMLEditor_statesType."Idle" ("state") UMLEditor_statesType."Repaint" ("state")] -> w4679
              tunnel: w4677 -> [_ w4692]
              tunnel: w4676 -> [_ w4691]
              tunnel: w4675 -> [_ w4690]
              frame 0, Default {
                n1811 = property on="Diagram" class="Ring (strict)"("Val(Sgnl)"=w4685) -> ()  [unwired: 2 in, 2 out]
              }
              frame -1 {
                n1812 = Strip Path(path=w4690) -> (stripped path=w4700:path, name=w4701:string)
                n1813 = call <resource>:"loadGraph.vi"("filePath"=w4690, "graphics"=w4691, "grid"=w4692, "error in (no error)"=w4689) -> ("reference out"=w4699:refnum<class "Graph.lvclass">, "succeeded"=w4702:bool, "diagramType"=w4695:T11, "NodesBounds"=w4693:T13, "error out"=w4703:errorcluster)  [unwired: 11 out]
                n1814 = case shown="True" w4702 {
                  tunnel: w4704 -> [w4706 w4736]
                  tunnel: w4703 -> [_ w4726]
                  tunnel: w4701 -> [_ w4739]
                  tunnel: w4700 -> [_ w4738]
                  tunnel: w4699 -> [_ w4707]
                  tunnel: w4695 -> [_ w4737]
                  tunnel: w4698 -> [_ w4734]
                  tunnel: [w4705 w4709] -> w4697
                  tunnel: w4690 -> [_ w4731]
                  tunnel: [w4706 w4714] -> w4696
                  tunnel: w4695 -> [_ w4715]
                  tunnel: w4690 -> [_ w4718]
                  tunnel: w4693 -> [_ w4713]
                  tunnel: w4689 -> [w4705 _]
                  frame False {
                  }
                  frame True {
                    n1815 = case shown="True" w4734 {
                      tunnel: w4726 -> [w4759 w4764]
                      tunnel: [w4760 w4763] -> w4721
                      tunnel: w4736 -> [w4760 w4762]
                      tunnel: [w4759 w4761] -> w4735
                      frame False {
                      }
                      frame True {
                        n1816 = call <resource>:"UMLEditor closeDiagram.vi"("error in (no error)"=w4764, "localVariablesIn"=w4762) -> ("localVariablesOut"=w4763:T7, "error out"=w4761:errorcluster)  [unwired: 16 out]
                      }
                    }
                    n1817 = Bundle By Name(cluster=w4721, "NodesBounds"=w4713, "toolType"=UMLEditor_tooltype."None", "selcted"=UMLEditor_tooltype."None") -> (w4722:T7)
                    n1818 = case shown="\"Class\", Default" w4715 {
                      tunnel: w4722 -> [w4741 w4745 w4749 w4754 w4758]
                      tunnel: [w4740 w4744 w4748 w4753 w4757] -> w4724
                      frame "None" {
                        n1819 = Bundle By Name(cluster=w4741, "tool"=UMLEditor_toolsType."CD_Select") -> (w4740:T7)
                      }
                      frame "Sequency" {
                        n1820 = Bundle By Name(cluster=w4745, "tool"=UMLEditor_toolsType."SQD_Select") -> (w4744:T7)
                        n1821 = property on="toolTab" class="TabCtl (strict)"("Value"=enum32{"Class", "Sequence", "UseCase"}."Sequence" ("toolTab")) -> ()  [unwired: 2 in, 2 out]
                      }
                      frame "UseCase" {
                        n1822 = Bundle By Name(cluster=w4749, "tool"=UMLEditor_toolsType."UD_Select") -> (w4748:T7)
                        n1823 = property on="toolTab" class="TabCtl (strict)"("Value"=enum32{"Class", "Sequence", "UseCase"}."UseCase" ("toolTab")) -> ()  [unwired: 2 in, 2 out]
                      }
                      frame "State" {
                        n1824 = Bundle By Name(cluster=w4754, "tool"=UMLEditor_toolsType."STD_Select") -> (w4753:T7)
                        n1825 = property on="toolTab" class="TabCtl (strict)"("Value"=enum32{"Class", "Sequence", "UseCase", "State"}."State" ("toolTab")) -> ()  [unwired: 2 in, 2 out]
                      }
                      frame "Class", Default {
                        n1826 = Bundle By Name(cluster=w4758, "tool"=UMLEditor_toolsType."CD_Select") -> (w4757:T7)
                        n1827 = property on="toolTab" class="TabCtl (strict)"("Value"=enum32{"Class", "Sequence", "UseCase"}."Class" ("toolTab")) -> ()  [unwired: 2 in, 2 out]
                      }
                    }
                    n1828 = Path To String(path=w4718) -> (string=w4719:string)
                    n1829 = property on="Diagram" class="Ring (strict)"("Tip Strip"=w4719) -> ()  [unwired: 2 in, 2 out]
                    n1830 = call <resource>:"UMLEditor addDiagram.vi"("graph"=w4707, "diagramType"=w4737, "name"=w4739, "saveDir"=w4738, "error in (no error)"=w4735, "localVariablesIn"=w4724) -> ("localVariablesOut"=w4714:T7, "error out"=w4733:errorcluster)  [unwired: 1 in, 11 out]
                    n1831 = Path To String(path=w4731) -> (string=w4730:string)
                    n1832 = Unbundle By Name(w4714) -> ("menu"=w4708:refnum<k9>)
                    n1833 = call <resource>:"UMLEditor menuUpdates.vi"("menu"=w4708, "menuAction"=UMLEditor_MenuActionType."AddRecentFile", "item"=w4730, "addfirst(false)"=TRUE, "error in (no error)"=w4733) -> ("error out"=w4729:errorcluster)  [unwired: 1 in, 13 out]
                    n1834 = call <resource>:"UMLEditor menuUpdates.vi"("menu"=w4708, "menuAction"=UMLEditor_MenuActionType."DiableSave", "error in (no error)"=w4729) -> ("error out"=w4716:errorcluster)  [unwired: 3 in, 13 out]
                    n1835 = property on="Picture" class="Pict"("Visible"=TRUE) -> ()  [unwired: 2 in, 2 out]
                    n1836 = property on="toolTab" class="TabCtl (strict)"("Disabled"=u8 0) -> ()  [unwired: 2 in, 2 out]
                    n1837 = call <resource>:"UMLEditor ToolsMenuUpdates.vi"("menu"=w4708, "diagramType"=w4715, "error in (no error)"=w4716) -> ("error out"=w4710:errorcluster)  [unwired: 3 in, 13 out]
                    n1838 = call <resource>:"UMLEditor UpdatesToolbuttons.vi"() -> ()  [unwired: 6 in, 14 out]
                    n1839 = call <resource>:"UndoEngine.vi"("reference"=w4707, "Action"=enum16{"TakeSnapshot", "Undo", "Redo"}."TakeSnapshot", "Reset"=TRUE, "error in (no error)"=w4710, "menu"=w4708) -> ("error out"=w4709:errorcluster)  [unwired: 3 in, 11 out]
                  }
                }
              }
            }
          }
        }
        n1840 = local write "Sync"(FALSE ("Sync")) -> ()
      }
      frame "Close" {
        w4765 = FALSE ("Sync")
        n1841 = call <resource>:"UMLEditor getDiagramInfo.vi"("localVariables"=w4767, "error in (no error)"=w4775) -> ("name"=w4773:string, "unsaved"=w4774:bool, "error out"=w4776:errorcluster)  [unwired: 15 out]
        n1842 = case shown="True" w4774 {
          tunnel: w4773 -> [_ w4845]
          tunnel: [FALSE ("Visible") w4844] -> w4772
          tunnel: w4769 -> [_ w4842]
          tunnel: [_ w4841] -> w4768
          frame False {
          }
          frame True {
            n1843 = Format Into String(format string="SAVE?\nYour work has not been saved!\nDo you want to save: %s", w4845) -> (resulting string=w4843:string)  [unwired: 2 in, 1 out]
            n1844 = case shown="Default" w4842 {
              tunnel: [w4850 w4858] -> w4844
              tunnel: w4843 -> [w4853 w4857]
              tunnel: [w4849 _] -> w4841
              frame "Exit" {
                n1845 = call <vilib>:"Three Button Dialog.vi"("Window Title (\"\")"="Save" ("Window Title (\"\")"), "Right Button Text (\"Cancel\")"="Don't quit" ("F button name (\"Cancel\")"), "Center Button Text (\"No\")"="Don't save" ("F button name (\"Cancel\")"), "Left Button Text (\"Yes\")"="Save" ("T button name (\"OK\")"), "message"=w4853) -> ("Which Button?"=w4848:T35)  [unwired: 6 out]
                n1846 = Greater Or Equal?(x=w4848, y=T35."Right Button") -> (x >= y?=w4849:bool)
                n1847 = Equal?(x=w4848, y=T35."Left Button") -> (x = y?=w4850:bool)
              }
              frame Default {
                n1848 = Two Button Dialog(message=w4857, 1:"Don't save" ("F button name (\"Cancel\")"), 2:"Save" ("T button name (\"OK\")")) -> (T button?=w4858:bool)
              }
            }
          }
        }
        n1849 = local write "Sync"(w4765) -> ()
        n1850 = Bundle By Name(cluster=w4767, "Sync"=w4765) -> (w4766:T7)
        n1851 = case shown="False" w4768 {
          tunnel: [w4783 w4835] -> w4777
          tunnel: w4776 -> [w4782 w4835]
          tunnel: w4772 -> [w4781 _]
          tunnel: [w4780 UMLEditor_statesType."Repaint" ("state")] -> w4771
          tunnel: w4766 -> [w4779 w4837]
          tunnel: [w4778 w4836] -> w4770
          frame False {
            n1852 = case shown="False" w4781 {
              tunnel: [w4794 w4834] -> w4783
              tunnel: w4779 -> [w4792 w4832]
              tunnel: w4782 -> [w4791 w4834]
              tunnel: [w4790 UMLEditor_statesType."Save" ("state")] -> w4780
              tunnel: [w4787 w4832] -> w4778
              frame False {
                n1853 = call <resource>:"UMLEditor closeDiagram.vi"("error in (no error)"=w4791, "localVariablesIn"=w4792) -> ("localVariablesOut"=w4785:T7, "lastDiagramClosed"=w4793:bool, "diagramType"=w4788:T11, "error out"=w4794:errorcluster)  [unwired: 14 out]
                n1854 = Bundle By Name(cluster=w4785, "toolType"=UMLEditor_tooltype."None") -> (w4786:T7)
                n1855 = Unbundle By Name(w4785) -> ("quit"=w4789:bool)
                n1856 = case shown="False" w4789 {
                  tunnel: w4793 -> [w4799 _]
                  tunnel: [w4798 UMLEditor_statesType."Exit" ("state")] -> w4790
                  tunnel: w4788 -> [w4797 _]
                  tunnel: w4786 -> [w4796 w4830]
                  tunnel: [w4795 w4830] -> w4787
                  frame False {
                    n1857 = case shown="False" w4799 {
                      tunnel: [UMLEditor_statesType."Repaint" ("state") UMLEditor_statesType."Idle" ("state")] -> w4798
                      tunnel: w4797 -> [w4802 _]
                      tunnel: w4796 -> [w4801 w4825]
                      tunnel: [w4800 w4824] -> w4795
                      frame False {
                        n1858 = case shown="\"State\"" w4802 {
                          tunnel: w4801 -> [w4805 w4809 w4813 w4817 w4822]
                          tunnel: [w4804 w4808 w4812 w4816 w4821] -> w4800
                          frame "None" {
                            n1859 = Bundle By Name(cluster=w4805, "tool"=UMLEditor_toolsType."CD_Select") -> (w4804:T7)
                          }
                          frame "Sequency" {
                            n1860 = Bundle By Name(cluster=w4809, "tool"=UMLEditor_toolsType."SQD_Select") -> (w4808:T7)
                            n1861 = property on="toolTab" class="TabCtl (strict)"("Value"=enum32{"Class", "Sequence", "UseCase"}."Sequence" ("toolTab")) -> ()  [unwired: 2 in, 2 out]
                          }
                          frame "UseCase" {
                            n1862 = Bundle By Name(cluster=w4813, "tool"=UMLEditor_toolsType."UD_Select") -> (w4812:T7)
                            n1863 = property on="toolTab" class="TabCtl (strict)"("Value"=enum32{"Class", "Sequence", "UseCase", "State"}."UseCase" ("toolTab")) -> ()  [unwired: 2 in, 2 out]
                          }
                          frame "State" {
                            n1864 = Bundle By Name(cluster=w4817, "tool"=UMLEditor_toolsType."STD_Select") -> (w4816:T7)
                            n1865 = property on="toolTab" class="TabCtl (strict)"("Value"=enum32{"Class", "Sequence", "UseCase", "State"}."State" ("toolTab")) -> ()  [unwired: 2 in, 2 out]
                          }
                          frame "Class", Default {
                            n1866 = Bundle By Name(cluster=w4822, "tool"=UMLEditor_toolsType."CD_Select") -> (w4821:T7)
                            n1867 = property on="toolTab" class="TabCtl (strict)"("Value"=enum32{"Class", "Sequence", "UseCase", "State"}."Class" ("toolTab")) -> ()  [unwired: 2 in, 2 out]
                          }
                        }
                      }
                      frame True {
                        n1868 = property on="toolTab" class="TabCtl (strict)"("Disabled"=u8 2) -> ()  [unwired: 2 in, 2 out]
                        n1869 = property on="Diagram" class="Ring (strict)"("Strings []"=string[] []) -> ()  [unwired: 2 in, 2 out]
                        n1870 = Bundle By Name(cluster=w4825, "tool"=UMLEditor_toolsType."SQD_Select") -> (w4824:T7)
                        n1871 = property on="Picture" class="Pict"("Visible"=FALSE) -> ()  [unwired: 2 in, 2 out]
                      }
                    }
                  }
                  frame True {
                  }
                }
                n1872 = call <resource>:"UMLEditor UpdatesToolbuttons.vi"() -> ()  [unwired: 6 in, 14 out]
              }
              frame True {
              }
            }
          }
          frame True {
            n1873 = Bundle By Name(cluster=w4837, "quit"=FALSE) -> (w4836:T7)
          }
        }
      }
      frame "CreateScript", "ExecuteScript" {
        n1874 = case shown="Default" w4874 {
          tunnel: w4880 -> [w4887 w4904]
          tunnel: [w4889 w4895] -> _
          tunnel: [w4888 w4903] -> _
          tunnel: w4878 -> [_ w4902]
          tunnel: w4877 -> [w4885 w4899]
          tunnel: [w4885 w4898] -> w4876
          tunnel: [w4886 w4897] -> w4879
          tunnel: [FALSE TRUE] -> _
          frame "ExecuteScript" {
            (unwired) T58."existing file" ("select mode (2)")
